vi "HEWH Gas Notifier.vi"(7 "Status":T2, 8 "error in (no error)":errorcluster, 10 "Gas Measurment Data":T1, 11 "name (unnamed)":string) -> (0 "error out":errorcluster, 3 "Gas Measurment Data Output":T1)   [LabVIEW 2019]
uses:
  Utility/Type Definitions/UTILITY Notifier.ctl
  Drivers/Alicat Gas Meter Driver/Sub-VIs/Data Cluster.ctl
panel:
  # "Totalizer Timer"
  # "Totalizer Timer"
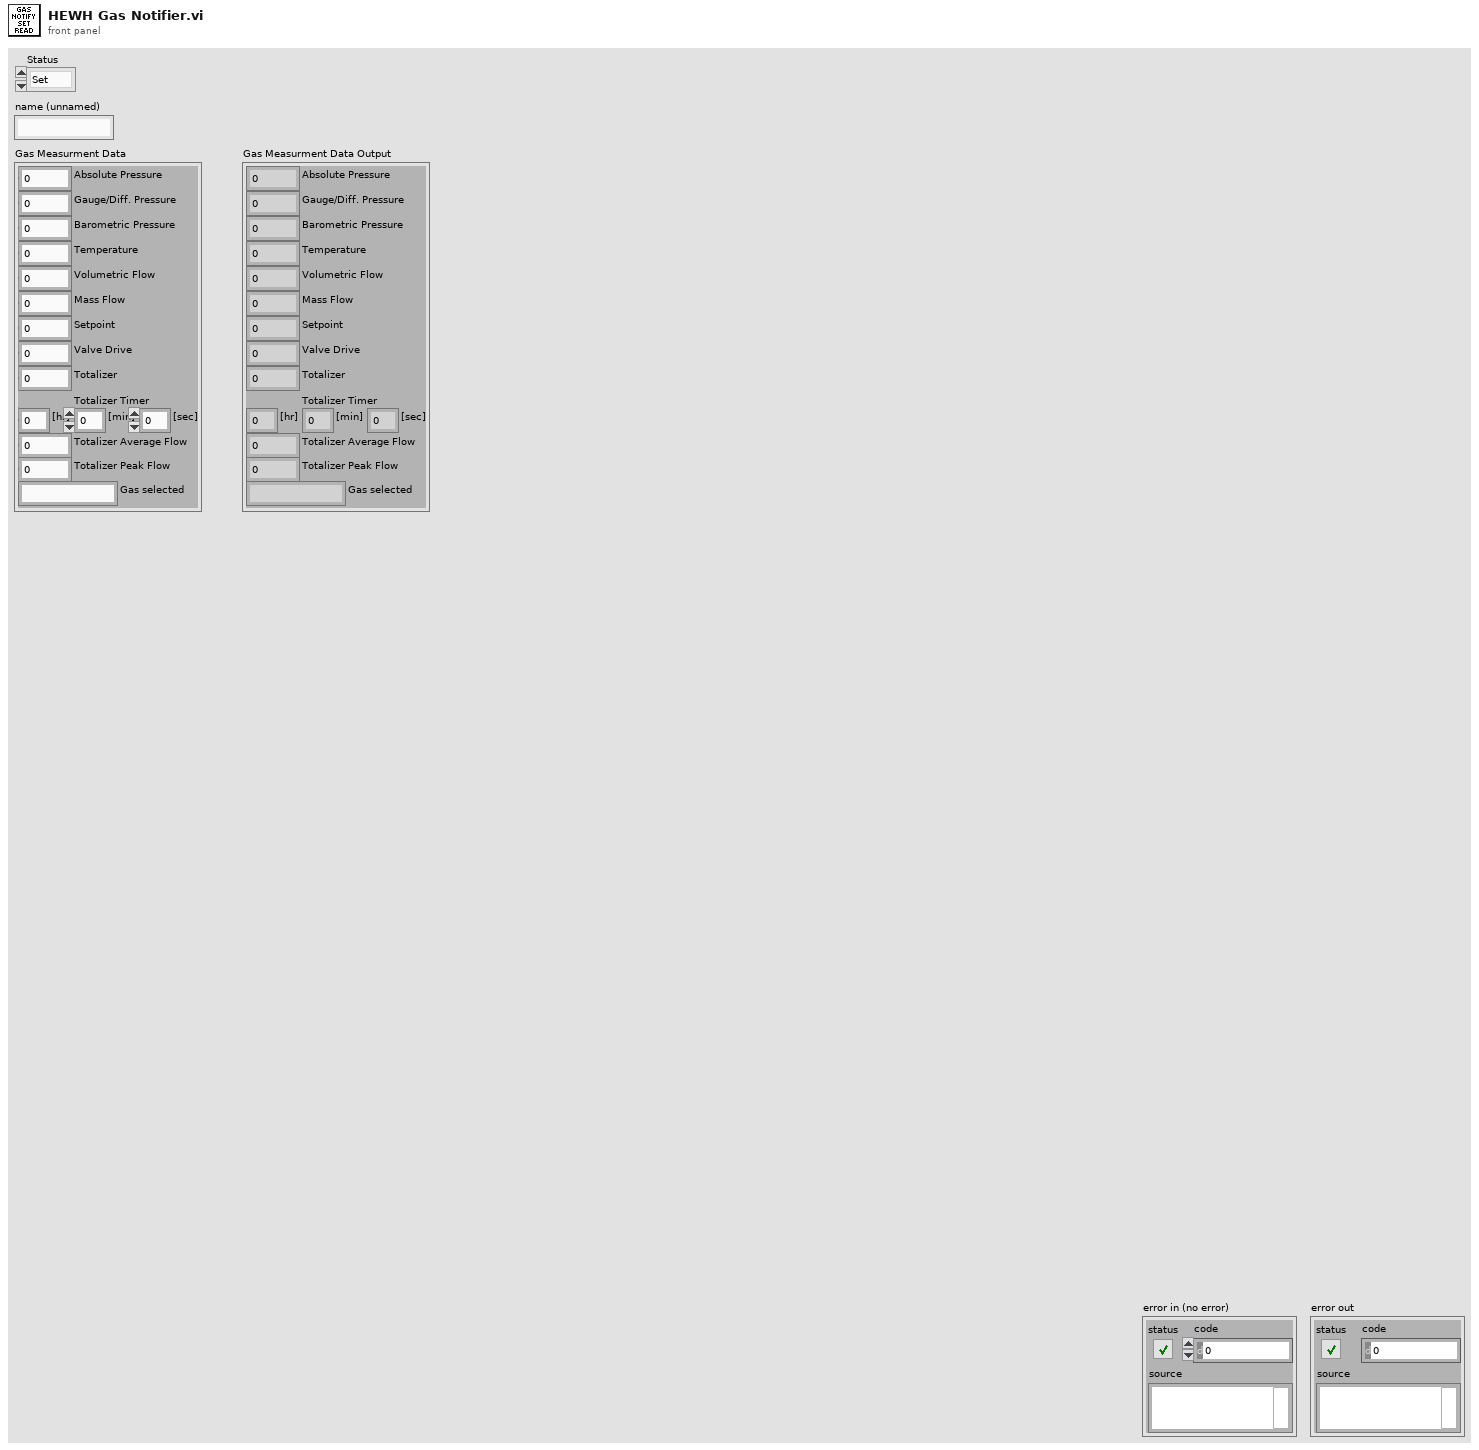
[diagram p1: front panel]
types:
  T1 = typedef "Data Cluster.ctl" = cluster{"Absolute Pressure":dbl, "Gauge/Diff. Pressure":dbl, "Barometric Pressure":dbl, "Temperature":dbl, "Volumetric Flow":dbl, "Mass Flow":dbl, "Setpoint":dbl, "Valve Drive":dbl, "Totalizer":dbl, "[hr]":dbl, "[min]":dbl, "[sec]":dbl, "Totalizer Average Flow":dbl, "Totalizer Peak Flow":dbl, "Gas selected":string}
  T2 = typedef "UTILITY Notifier.ctl" = enum16{"Set", "Read", "Release Ref"}
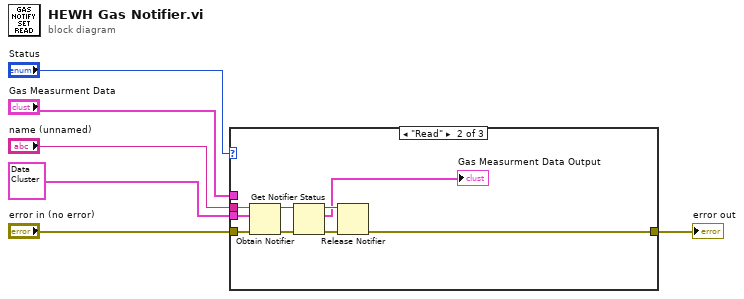
[diagram p0: block diagram]
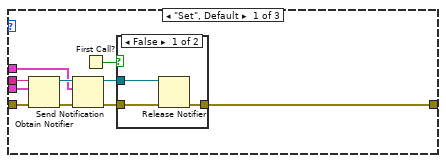
[diagram p2: hidden frame]
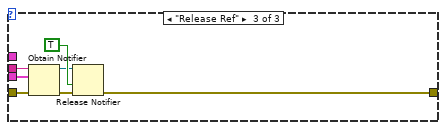
[diagram p4: hidden frame]
diagram:
  n1 = case shown="\"Read\"" "Status" {
    tunnel: [w7 w23 w32] -> w6
    tunnel: "error in (no error)" -> [w14 w27 w33]
    tunnel: "name (unnamed)" -> [w13 w26 w31]
    tunnel: T1 {"Absolute Pressure"=0.0, "Gauge/Diff. Pressure"=0.0, "Barometric Pressure"=0.0, "Temperature"=0.0, "Volumetric Flow"=0.0, "Mass Flow"=0.0, "Setpoint"=0.0, "Valve Drive"=0.0, "Totalizer"=0.0, "[hr]"=0.0, "[min]"=0.0, "[sec]"=0.0, "Totalizer Average Flow"=0.0, "Totalizer Peak Flow"=0.0, "Gas selected"=""} ("Gas Measurment Data") -> [w11 w25 w30]
    tunnel: "Gas Measurment Data" -> [w12 _ _]
    frame "Set", Default {
      n2 = Obtain Notifier(name (unnamed)=w13, notification data type=w11, error in (no error)=w14) -> (notifier out=w15:refnum<notifier>, error out=w16:errorcluster)  [unwired: 1 in, 1 out]
      n3 = Send Notification(notification=w12, notifier=w15, error in (no error)=w16) -> (notifier out=w9:refnum<notifier>, error out=w10:errorcluster)
      n4 = First Call?() -> (First Call?: T/F=w8:bool)
      n5 = case shown="False" w8 {
        tunnel: w10 -> [w19 w20]
        tunnel: [w18 w20] -> w7
        tunnel: w9 -> [w17 _]
        frame False {
          n6 = Release Notifier(notifier=w17, error in (no error)=w19) -> (error out=w18:errorcluster)  [unwired: 1 in, 2 out]
        }
        frame True {
        }
      }
    }
    frame "Read" {
      n7 = Obtain Notifier(name (unnamed)=w26, notification data type=w25, error in (no error)=w27) -> (notifier out=w28:refnum<notifier>, error out=w29:errorcluster)  [unwired: 1 in, 1 out]
      n8 = Get Notifier Status(notifier=w28, error in (no error)=w29) -> (notifier out=w22:refnum<notifier>, current notification=→"Gas Measurment Data Output":T1, error out=w24:errorcluster)  [unwired: 2 out]
      n9 = Release Notifier(notifier=w22, error in (no error)=w24) -> (error out=w23:errorcluster)  [unwired: 1 in, 2 out]
    }
    frame "Release Ref" {
      n10 = Obtain Notifier(name (unnamed)=w31, notification data type=w30, error in (no error)=w33) -> (notifier out=w35:refnum<notifier>, error out=w34:errorcluster)  [unwired: 1 in, 1 out]
      n11 = Release Notifier(notifier=w35, force destroy? (F)=TRUE, error in (no error)=w34) -> (error out=w32:errorcluster)  [unwired: 2 out]
    }
  }
  "error out" <- w6
